vi "SP Unpack and Check Stimulus.vi"(3 "Flat Stimulus":string, 5 "Requested Stimulus In":T1 {"Sweep Time (s)" format="%.3g"}) -> (0 "Stimulus Changed?":bool, 1 "Current Stimulus":T1 {"Sweep Time (s)" format="%.3g"}, 2 "Requested Stimulus Out":T1 {"Sweep Time (s)" format="%.3g"})   [LabVIEW 2011]
uses:
  TypeDefs/SP Stimulus Parameters.ctl
  TypeDefs/SP Frequency Units.ctl
  TypeDefs/SP Calibration State.ctl
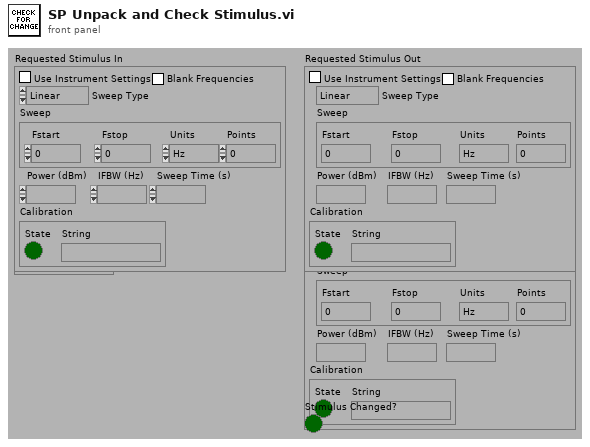
[diagram p1: front panel]
types:
  T1 = typedef "SP Stimulus Parameters.ctl" = cluster{"Use Instrument Settings":bool, "Blank Frequencies":bool, "Sweep Type":enum32{"Linear", "Logarithmic", "List", "Power", "CW"}, "Sweep":cluster{"Fstart":dbl, "Fstop":dbl, "Units":T2, "Points":i32}, "Power (dBm)":dbl, "IFBW (Hz)":dbl, "Sweep Time (s)":dbl, "Calibration":T3}
  T2 = typedef "SP Frequency Units.ctl" = enum16{"Hz", "kHz", "MHz", "GHz", "Points"}
  T3 = typedef "SP Calibration State.ctl" = cluster{"State":bool, "String":string}
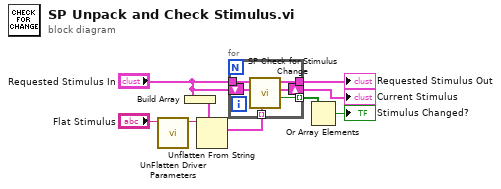
[diagram p0: block diagram]
diagram:
  n1 = call "UnFlatten Driver Parameters.vi"("Flattened Driver Parameters with Version (\"\")"="Flat Stimulus") -> ("Flat Driver Parameters"=w1:string)  [unwired: 1 in, 5 out]
  n2 = Build Array("Requested Stimulus In") -> (w4:T1[])
  n3 = Unflatten From String(type=w4, binary string=w1) -> (value=w7:T1[])  [unwired: 1 in, 4 out]
  n4 = for {
    tunnel: [w15] -> w2 mode=indexing
    tunnel: [w12] -> w3
    tunnel: w7 -> [w14] mode=indexing
    tunnel: "Requested Stimulus In" -> [w13]
    shift-right: [w10] -> w8
    shift-left: "Requested Stimulus In" -> [w11]
    n5 = call "SP Check for Stimulus Change.vi"("Current Stimulus Channel"=w14, "Current Stimulus In"=w11, "New Stimulus"=w13) -> ("Stimulus Changed?"=w15:bool, "Current Stimulus Out"=w10:T1, "Stimulus to Set"=w12:T1)  [unwired: 6 out]
  }
  "Current Stimulus" <- w8
  "Requested Stimulus Out" <- w3
  n6 = Or Array Elements(Boolean array=w2) -> (logical OR=→"Stimulus Changed?":bool)
